vi "Read Averaging time.vi"(8 "error in (no error)":errorcluster, 11 "RP Lockin in":refnum<class "RP Transceiver.lvclass">) -> (0 "error out":errorcluster, 2 "Time constant":dbl, 3 "RP Lockin out":refnum<class "RP Transceiver.lvclass">)   [LabVIEW 2016, in "RP Transceiver.lvclass"]
uses:
  RP Transceiver.lvclass
  RP Transceiver.lvclass/RP Transceiver.ctl
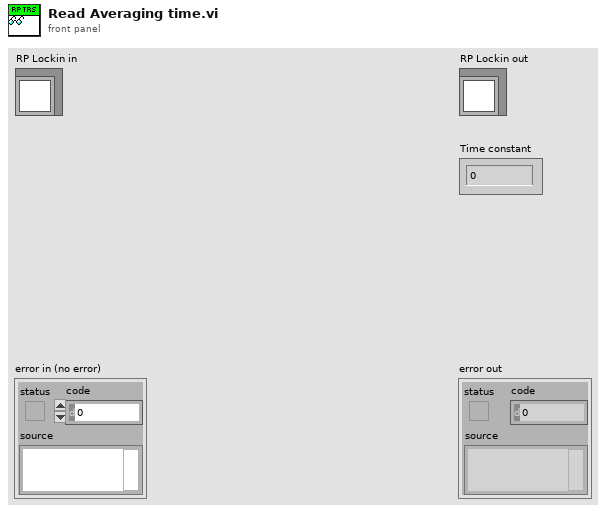
[diagram p1: front panel]
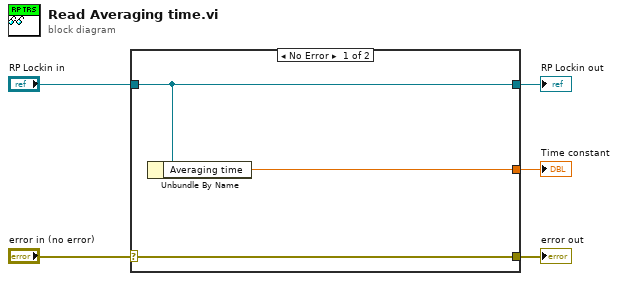
[diagram p0: block diagram]
diagram:
  n1 = case shown="No Error" "error in (no error)" {
    selector: "error in (no error)" -> [w8 w9]
    tunnel: [w8 w9] -> w4
    tunnel: [w7 w10] -> w2
    tunnel: "RP Lockin in" -> [w7 w10]
    tunnel: [w6 _] -> w1
    frame No Error {
      n2 = Unbundle By Name(w7) -> ("Averaging time"=w6:dbl)
    }
    frame Error {
    }
  }
  "error out" <- w4
  "RP Lockin out" <- w2
  "Time constant" <- w1
